vi "Create.vi"(8 "error in (no error)":errorcluster) -> (0 "error out":errorcluster, 3 "DAQ Data":refnum<data-value>)   [LabVIEW 2022 SP3, in "DAQ Data.lvclass"]
uses:
  DAQ Data.lvclass
  DAQ Data.lvclass/DAQ Data.ctl
  Events.ctl
  AIDAQ Data.ctl
  AI Daq Data.lvlib
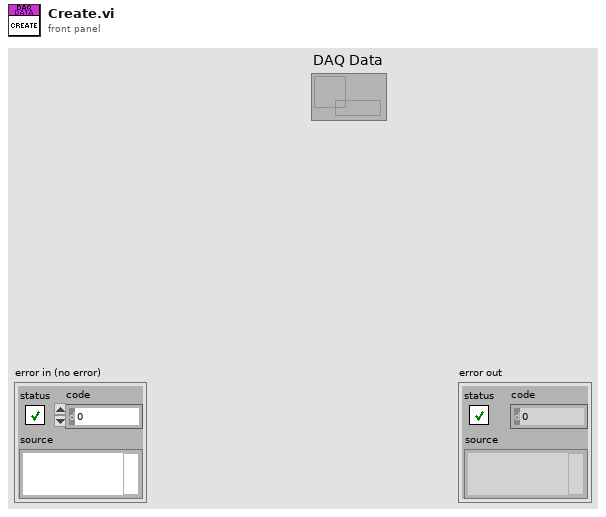
[diagram p1: front panel]
types:
  T1 = typedef "DAQ Data.lvclass/Events.ctl" = cluster{"AI Data":refnum<user-event>, "AI Channel Data":refnum<user-event>}
  T2 = typedef "AI Daq Data.lvlib/AIDAQ Data.ctl" = cluster{"AI":dbl, "Time Stamp":timestamp}
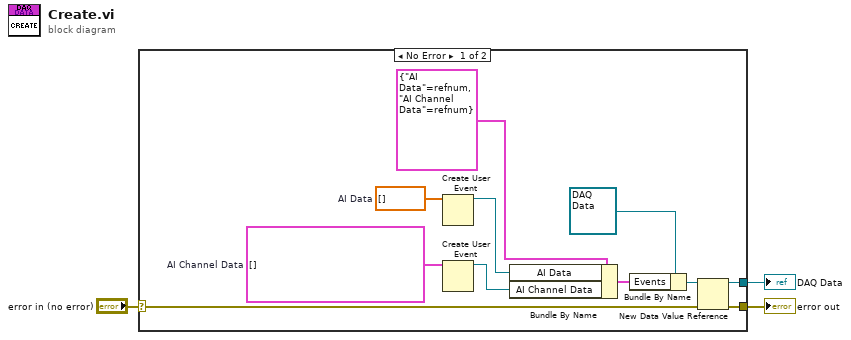
[diagram p0: block diagram]
diagram:
  n1 = case shown="No Error" "error in (no error)" {
    selector: "error in (no error)" -> [w6 w15]
    tunnel: [w5 w15] -> w2
    tunnel: [w13 _] -> w1
    frame No Error {
      w4 = cluster{"AI Channel Data":T2[]}[] []  # AI Channel Data
      w12 = dbl[] []  # AI Data
      n2 = Create User Event(user event datatype=w12) -> (user event=w10:refnum<user-event>)  [unwired: 1 in, 1 out]
      n3 = Create User Event(user event datatype=w4) -> (user event=w9:refnum<user-event>)  [unwired: 1 in, 1 out]
      n4 = Bundle By Name(cluster=T1 {"AI Data"=refnum, "AI Channel Data"=refnum} ("Events"), "AI Data"=w10, "AI Channel Data"=w9) -> (w7:T1)
      n5 = Bundle By Name(cluster=refnum<class "DAQ Data.lvclass"> refnum ("DAQ Data in"), "Events"=w7) -> (w8:refnum<class "DAQ Data.lvclass">)
      n6 = New Data Value Reference(data value=w8, error in=w6) -> (data value reference=w13:refnum<data-value>, error out=w5:errorcluster)
    }
    frame Error {
    }
  }
  "error out" <- w2
  "DAQ Data" <- w1
